vi "主画面.vi"() -> ()   [LabVIEW 2016]
uses:
  <vilib>/Utility/config.llb/Read Key (String).vi
  <vilib>/Utility/config.llb/NI_LVConfig.lvlib
  data/FreeMem.dll
panel:
  in  "全屏":bool
  out "站点名称":string="站点名称"
  in  "主画面菜单":enum32{"首页", "数据查询", "运维调试", "系统设置"}(xcontrol)
  out "时间显示":string="2017-05-09 10:50:42"
  out "Version":string="Version:1.0.0"
  # "一体化微 型 水 质 监 测 站"
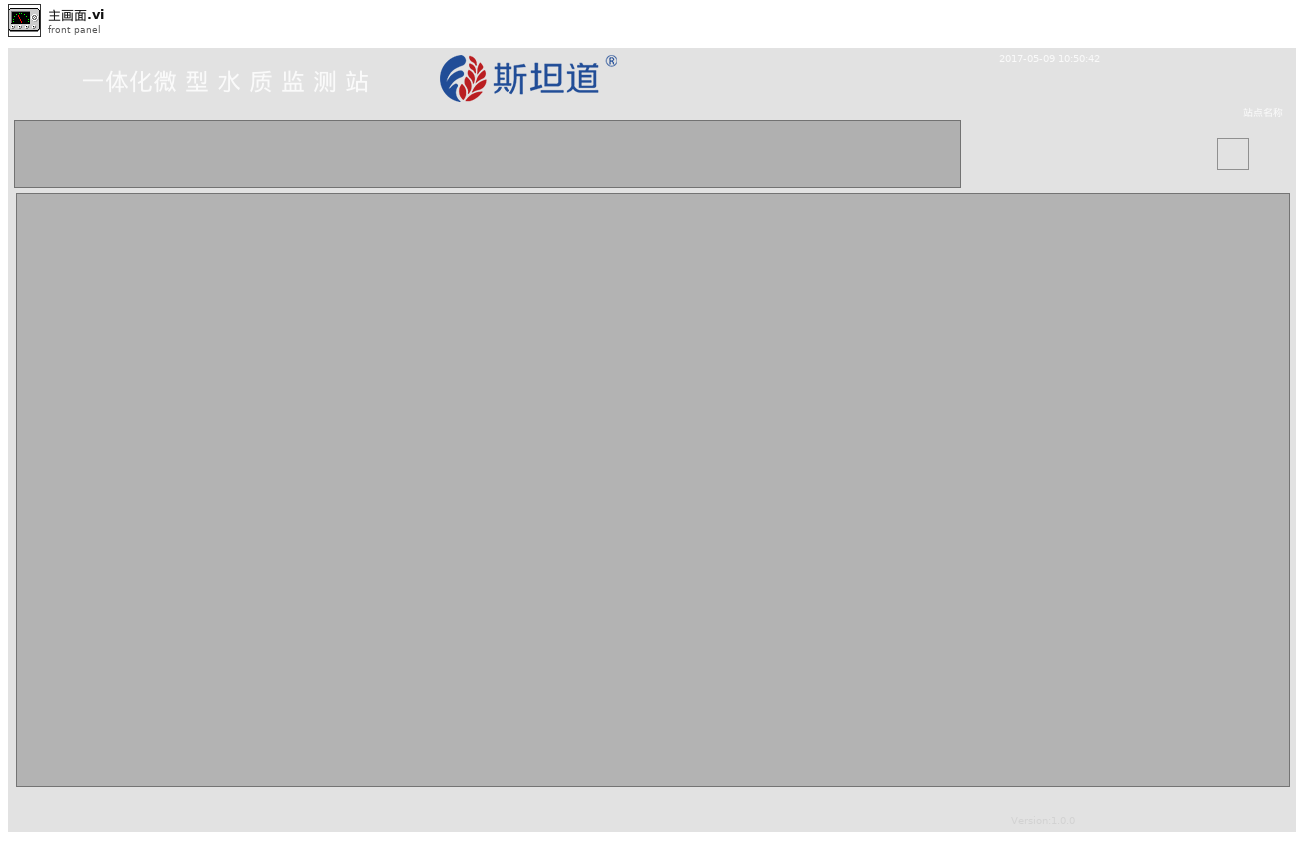
[diagram p1: front panel]
types:
  T1 = enum32{"invalid app kind", "Development System", "Run Time System", "Student Edition", "Embedded LabVIEW", "Evaluation", "Custom"}
  T2 = typedef "NI_LVConfig.lvlib/Config Data RefNum.ctl" = refnum<k1>
  T3 = enum32{"Bad", "Idle", "Run top level", "Running"}
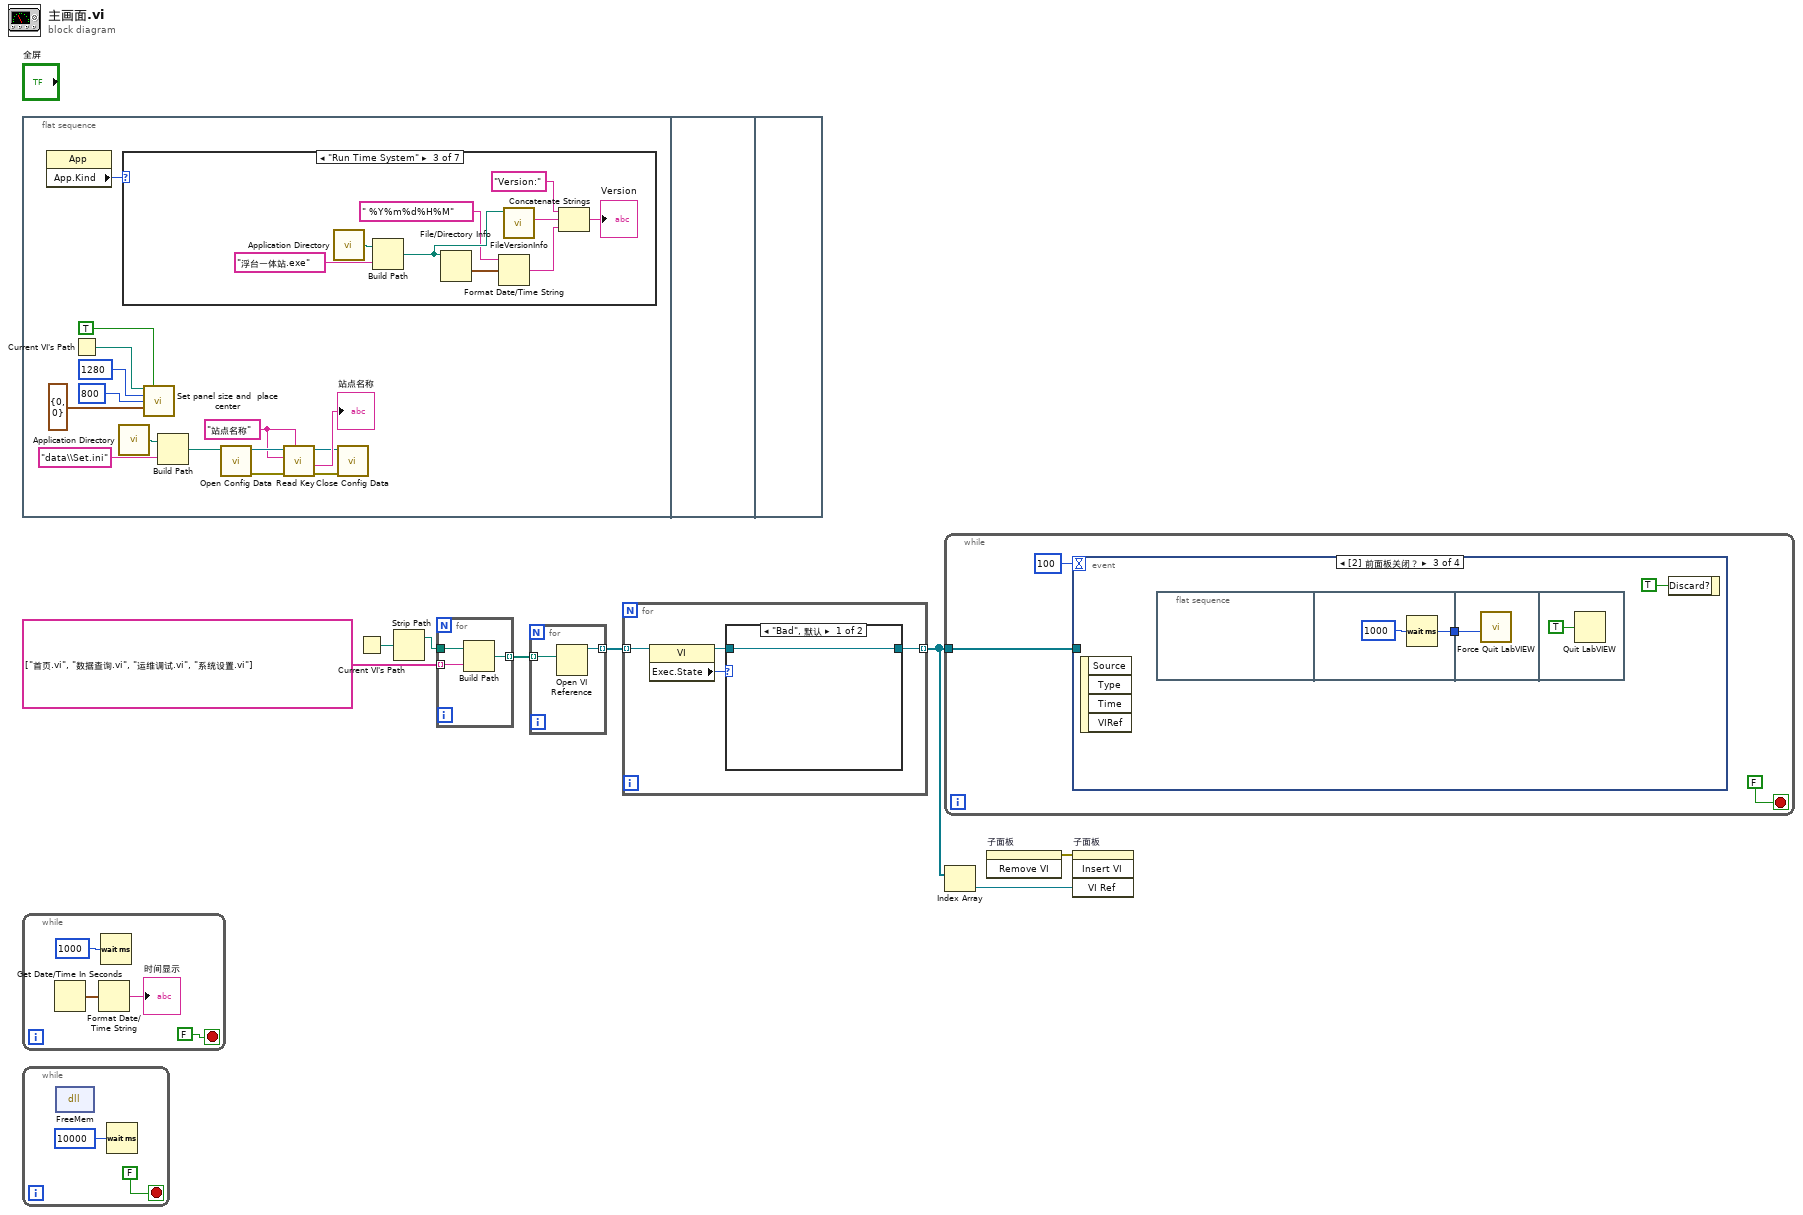
[diagram p0: block diagram]
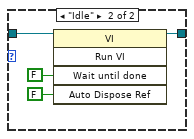
[diagram p2: hidden frame]
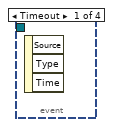
[diagram p9: hidden frame]
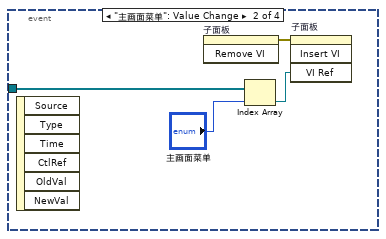
[diagram p10: hidden frame]
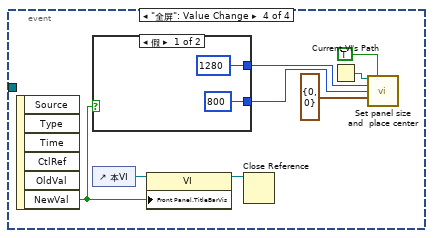
[diagram p11: hidden frame]
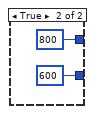
[diagram p12: hidden frame]
diagram:
  n1 = flat-sequence {
    frame #0 {
      w9 = "站点名称" ("section")
      n2 = property class="App"() -> ("App.Kind"=w20:T1)  [unwired: 2 in, 2 out]
      n3 = Current VI's Path() -> (path=w23:path)
      n4 = call <vilib>:"Application Directory.vi"() -> ("Application Directory"=w12:path)
      n5 = case shown="\"Run Time System\"" w20 {
        frame "invalid app kind" {
        }
        frame "Development System", Default {
        }
        frame "Run Time System" {
          n6 = call <vilib>:"Application Directory.vi"() -> ("Application Directory"=w31:path)
          n7 = Build Path(base path=w31, name or relative path="浮台一体站.exe" ("名称或相对路径")) -> (appended path=w27:path)
          n8 = File/Directory Info(path=w27) -> (last mod=w26:timestamp)  [unwired: 1 in, 6 out]
          n9 = Format Date/Time String(time format string (%c)=" %Y%m%d%H%M" ("时间格式字符串(%c)"), seconds (now)=w26) -> (date/time string=w24:string)  [unwired: 1 in]
          n10 = call <vilib>:"FileVersionInfo.vi"("Application Path in"=w27) -> ("File Version Info"=w29:string)  [unwired: 7 in, 3 out]
          n11 = Concatenate Strings("Version:" ("字符串"), w29, w24) -> (→"Version":string)
        }
        frame "Student Edition" {
        }
        frame "Embedded LabVIEW" {
        }
        frame "Evaluation" {
        }
        frame "Custom" {
        }
      }
      n12 = call "Set panel size and  place center.vi"("Path"=w23, "Close Reference (false)"=TRUE, "Panel Width"=1280, "Panel Height"=800, "FP.Origin in(H & V)"=cluster{"Horizontal":i16, "Vertical":i16} {"Horizontal"=0, "Vertical"=0}) -> ()  [unwired: 6 in, 5 out]
      n13 = Build Path(base path=w12, name or relative path="data\\Set.ini" ("名称或相对路径")) -> (appended path=w10:path)
      n14 = call <vilib>:"Open Config Data.vi"("configuration file path"=w10) -> ("error out"=w14:errorcluster, "refnum"=w17:T2)  [unwired: 8 in, 1 out]
      n15 = call-poly <vilib>:"Read Key.vi"("section"=w9, "error in (no error)"=w14, "key"=w9, "refnum"=w17) -> ("error out"=w13:errorcluster, "value"=→"站点名称":string, "refnum out"=w15:T2)  [unwired: 4 in, 1 out]
      n16 = call <vilib>:"Close Config Data.vi"("error in (no error)"=w13, "refnum"=w15) -> ()  [unwired: 8 in, 2 out]
    }
    frame #1 {
    }
    frame #2 {
    }
  }
  n17 = while {
    stop <- FALSE stop-if-true
    n18 = Get Date/Time In Seconds() -> (seconds since 1Jan1904=w33:timestamp)
    n19 = Format Date/Time String(seconds (now)=w33) -> (date/time string=→"时间显示":string)  [unwired: 2 in]
    n20 = Wait (ms)(milliseconds to wait=u32 1000 ("等待时间（毫秒）")) -> ()  [unwired: 1 out]
  }
  n21 = while {
    stop <- FALSE stop-if-true
    n22 = dll-call lib="PTH2Zabs CUserslisha\nSynologyDriveDrive项目集成环保认证dataFreeMem.dll" fn="FreeMem"() -> ()  [unwired: 4 in, 2 out]
    n23 = Wait (ms)(milliseconds to wait=u32 10000 ("等待时间（毫秒）")) -> ()  [unwired: 1 out]
  }
  n24 = Current VI's Path() -> (path=w8:path)
  n25 = Strip Path(path=w8) -> (stripped path=w7:path)  [unwired: 1 out]
  n26 = for {
    tunnel: w7 -> [w41]
    tunnel: string[] ["首页.vi", "数据查询.vi", "运维调试.vi", "系统设置.vi"] -> [w40] mode=indexing
    tunnel: [w39] -> w5 mode=indexing
    n27 = Build Path(base path=w41, name or relative path=w40) -> (appended path=w39:path)
  }
  n28 = for {
    tunnel: w5 -> [w43] mode=indexing
    tunnel: [w42] -> w4 mode=indexing
    n29 = Open VI Reference(vi path=w43) -> (vi reference=w42:refnum<vi>)  [unwired: 5 in, 1 out]
  }
  n30 = for {
    tunnel: w4 -> [w47] mode=indexing
    tunnel: [w44] -> w2 mode=indexing
    n31 = property class="VI"(reference=w47) -> (reference out=w45:refnum<vi>, "Exec.State"=w46:T3)  [unwired: 1 in, 1 out]
    n32 = case shown="\"Bad\", 默认" w46 {
      tunnel: w45 -> [w48 w50]
      tunnel: [w48 w49] -> w44
      frame "Bad", Default {
      }
      frame "Idle" {
        n33 = invoke class="VI" method="Run VI"(reference=w50, "Wait until done"=FALSE ("结束前等待"), "Auto Dispose Ref"=FALSE ("自动销毁引用")) -> (reference out=w49:refnum<vi>)  [unwired: 2 in, 4 out]
      }
    }
  }
  n34 = while {
    tunnel: w2 -> [w53]
    stop <- FALSE stop-if-true
    n35 = event shown="[2] 前面板关闭？" {
      selector: _ -> [_ _ _ _]
      dyn-events: _ -> [_ _ _ _]
      timeout: 100 -> [_ _ _ _]
      tunnel: w53 -> [_ w58 _ _]
      event Timeout {
        n36 = event-data() -> ()  [unwired: 1 in, 3 out]
      }
      event "主画面菜单": Value Change {
        n37 = event-data() -> ()  [unwired: 1 in, 6 out]
        n38 = invoke on="子面板" class="SubPnl" method="Remove VI"() -> (error out=w56:errorcluster)  [unwired: 3 in, 2 out]
        n39 = Index Array(array=w58, index="主画面菜单") -> (element=w57:refnum<vi>)
        n40 = invoke on="子面板" class="SubPnl" method="Insert VI"(error in=w56, "VI Ref"=w57) -> ()  [unwired: 2 in, 4 out]
      }
      event Panel Close? {
        n41 = event-data() -> ()  [unwired: 1 in, 4 out]
        n42 = flat-sequence {
          tunnel: [w63] -> w60
          tunnel: w60 -> [w64]
          frame #0 {
          }
          frame #1 {
            n43 = Wait (ms)(milliseconds to wait=u32 1000 ("等待时间（毫秒）")) -> (millisecond timer value=w63:u32)
          }
          frame #2 {
            n44 = call "Force Quit LabVIEW.vi"("Exit Code (0)"=w64) -> ()  [unwired: 9 in, 2 out]
          }
          frame #3 {
            n45 = Quit LabVIEW(quit? (T)=TRUE ("退出？(T)")) -> ()
          }
        }
        n46 = event-data("Discard?"=TRUE ("放弃？")) -> ()  [unwired: 1 in, 1 out]
      }
      event "全屏": Value Change {
        n47 = event-data() -> ("NewVal"=w71:bool)  [unwired: 1 in, 5 out]
        n48 = case shown="假" w71 {
          tunnel: [1280 ("Panel Width") 800 ("Panel Width")] -> w67
          tunnel: [800 ("Panel Height") 600 ("Panel Height")] -> w66
          frame False {
          }
          frame True {
          }
        }
        n49 = control-ref of="本VI"() -> (w72:refnum<vi>)
        n50 = property class="VI"(reference=w72, "Front Panel.TitleBarVis"=w71) -> (reference out=w73:refnum<vi>)  [unwired: 1 in, 1 out]
        n51 = Close Reference(reference=w73) -> ()  [unwired: 1 in, 1 out]
        n52 = Current VI's Path() -> (path=w70:path)
        n53 = call "Set panel size and  place center.vi"("Path"=w70, "Close Reference (false)"=TRUE, "Panel Width"=w67, "Panel Height"=w66, "FP.Origin in(H & V)"=cluster{"Horizontal":i16, "Vertical":i16} {"Horizontal"=0, "Vertical"=0}) -> ()  [unwired: 6 in, 5 out]
      }
    }
  }
  n54 = Index Array(array=w2) -> (element=w1:refnum<vi>)  [unwired: 1 in]
  n55 = invoke on="子面板" class="SubPnl" method="Remove VI"() -> (error out=w3:errorcluster)  [unwired: 3 in, 2 out]
  n56 = invoke on="子面板" class="SubPnl" method="Insert VI"(error in=w3, "VI Ref"=w1) -> ()  [unwired: 2 in, 4 out]
